vi "main.vi"(8 "Aantal frames":i32) -> (0 "Xhoek, Yafstand":dbl[](array[numeric]))   [LabVIEW 2021]
doc: "This example demonstrates how to call a Python function and pass integers as arguments. It uses a python function to compute the sum of two integers."
uses:
  Program Files (x86)/National Instruments/LabVIEW 2021/examples/Connectivity/Python/support/PythonVersionsEnum.ctl
panel:
  out "error out":errorcluster
  in  "error in (no error)":errorcluster
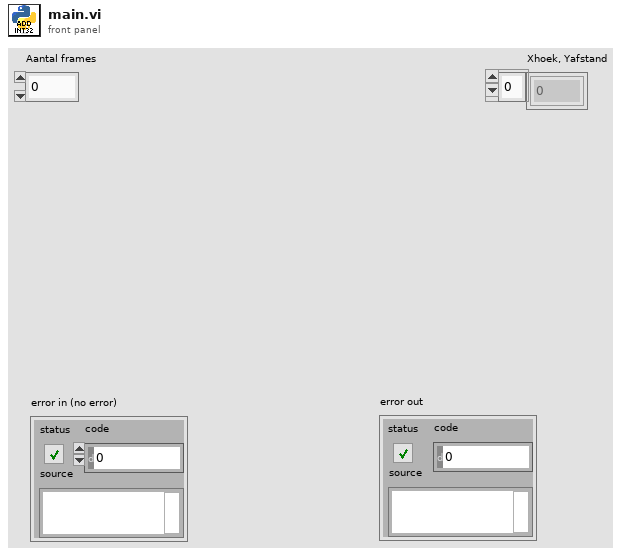
[diagram p1: front panel]
types:
  T1 = typedef "PythonVersionsEnum.ctl" = enum16{"3.6", "3.7", "3.8", "3.9"}
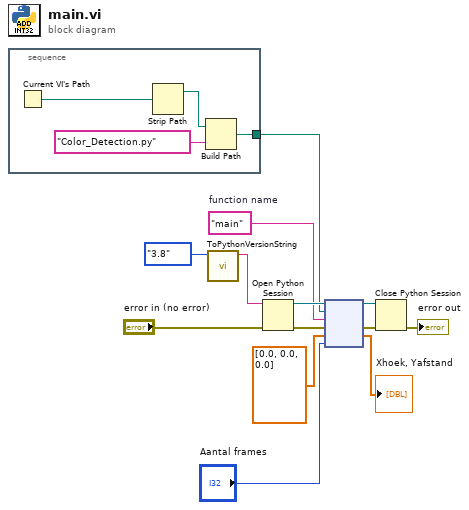
[diagram p0: block diagram]
diagram:
  w9 = "main"  # function name
  n1 = stacked-sequence {
    tunnel: [w17] -> w10
    frame #0 {
      n2 = Current VI's Path() -> (path=w14:path)
      n3 = Strip Path(path=w14) -> (stripped path=w15:path)  [unwired: 1 out]
      n4 = Build Path(base path=w15, name or relative path="Color_Detection.py") -> (appended path=w17:path)
    }
  }
  n5 = call "ToPythonVersionString.vi"("python version"=PythonVersionsEnum."3.8") -> ("python version string"=w5:string)  [unwired: 10 in]
  n6 = Open Python Session(python version=w5, 3:"error in (no error)") -> (session out=w12:refnum<k35>, error out=w11:errorcluster)  [unwired: 1 in]
  n7 = node(w12, w10, w9, w11, dbl[] [0.0, 0.0, 0.0], "Aantal frames") -> (w8:refnum<k35>, w7:errorcluster, →"Xhoek, Yafstand":dbl[])  [unwired: 1 in, 2 out]
  n8 = Close Python Session(session in=w8, error in=w7) -> (11:→"error out":errorcluster)
